vi "数据写入database.vi"(9 "data":variant, 10 "columns":string[](array[string]), 11 "table":string) -> (1 "error out":errorcluster)   [LabVIEW 2016, in "斯坦道CODMn.lvlib"]
uses:
  <vilib>/Utility/sysdir.llb/System Directory Type.ctl
  <vilib>/Utility/error.llb/DialogType.ctl
  <vilib>/addons/database/Auxilliary.llb/DB Tools Transaction.ctl
  <vilib>/addons/database/Auxilliary.llb/DB Tools Isolation Level.ctl
  <vilib>/addons/database/Connection.llb/DB Tools Open Connec (String).vi
  <vilib>/addons/database/Connection.llb/Conn Execute.vi
  <vilib>/addons/database/Recordset.llb/Rec Destroy - Connection.vi
  <vilib>/addons/database/Recordset.llb/Rec Fetch Recordset Data (R).vi
  <vilib>/addons/database/Connection.llb/Conn Transaction.vi
  <vilib>/addons/database/NI_Database_API.lvlib
panel:
  out "为空？":bool
  in  "error in (no error)":errorcluster
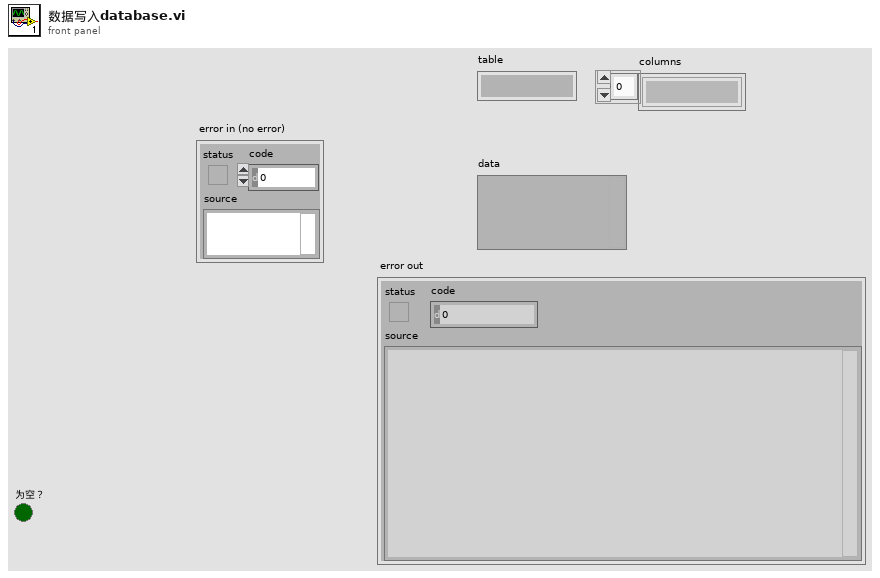
[diagram p1: front panel]
types:
  T1 = cluster{"时间":timestamp, "测量模式":string, "数据类型":string, "检测值":sgl, "单位":string, "数据标识":string, "因子编码":string, "标样参考值":sgl, "ORP-A":sgl, "ORP-B":sgl, "ORP-K":sgl, "COD滴定值":sgl, "高锰酸钾滴定数":sgl, "温度":sgl, "量程":sgl, "LastTime":timestamp, "序列号:":string}
  T2 = typedef "DialogType.ctl" = u16
  T3 = typedef "System Directory Type.ctl" = i32
  T4 = typedef "NI_Database_API.lvlib/Conn ObjectReference.ctl" = refnum<k1>
  T5 = typedef "NI_Database_API.lvlib/Rec ObjectReference.ctl" = refnum<k1>
  T6 = typedef "NI_Database_API.lvlib/DB Tools Transaction.ctl" = enum16{"begin", "commit", "rollback"}
  T7 = typedef "NI_Database_API.lvlib/DB Tools Isolation Level.ctl" = enum16{"chaos", "read uncommitted", "read committed", "repeatable read", "serializable"}
  T8 = cluster{"测量量程":dbl, "测量精度":dbl, "测量间隔":dbl, "消解温度":dbl, "消解时长":dbl, "空白校准时间":timestamp, "曲线截距":dbl, "曲线斜率":dbl, "测量检出限":dbl, "测量信号值":dbl, "线性相关系数":dbl, "二次多项式系数":dbl, "标样校准时间":timestamp, "稀释倍数":dbl, "三项式系数":dbl, "空白标定系数":dbl, "量程系数":dbl, "F0/ORPA":dbl, "F1/ORPB":dbl, "F2/ORPK":dbl, "F3":dbl, "F4":dbl, "F5":dbl, "F6":dbl, "F7":dbl, "X0/滴定数":dbl, "量程":dbl}
  T9 = cluster{"时间标识":timestamp, "设备":string, "日志信息":string}
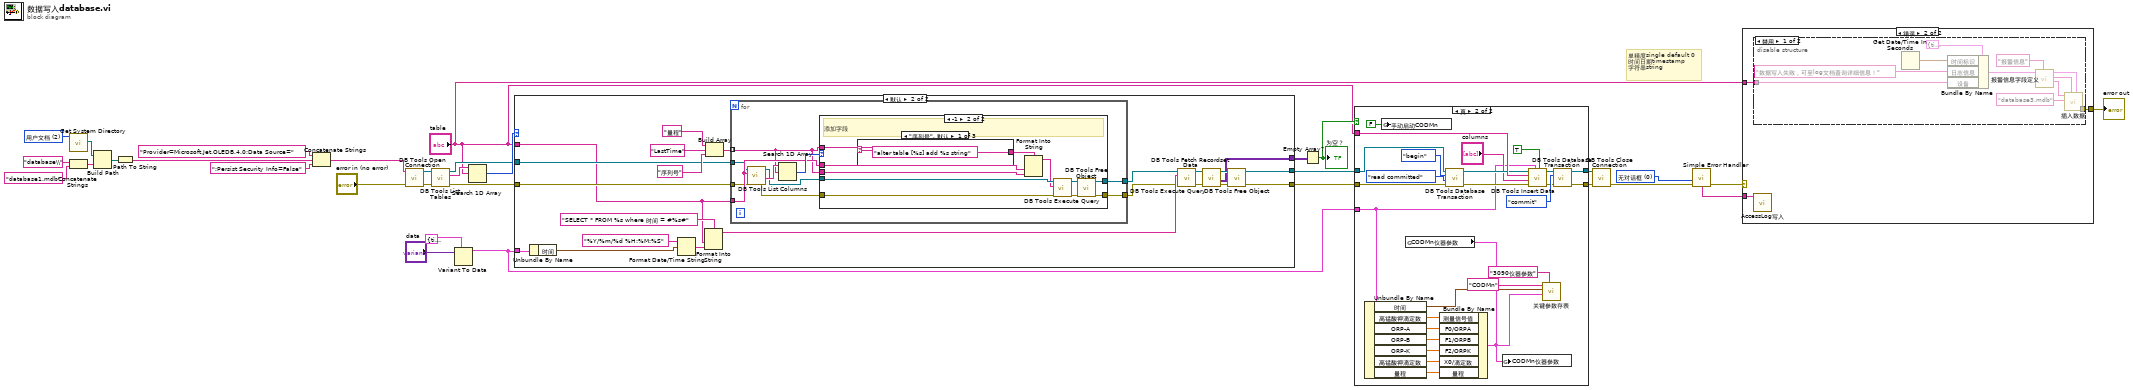
[diagram p0: block diagram]
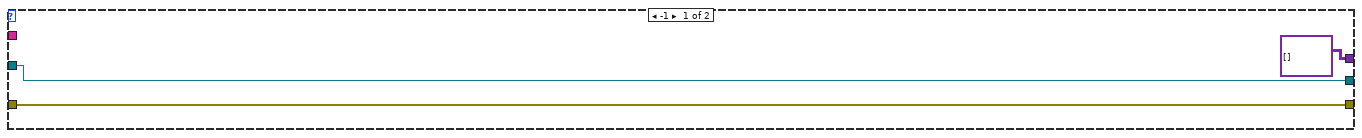
[diagram p4: hidden frame]
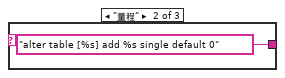
[diagram p6: hidden frame]
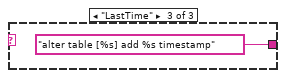
[diagram p7: hidden frame]
diagram:
  w8 = T2 0 items=["无对话框", "确定信息", "继续或停止信息", "确定信息＋警告", "继续/停止+警告"] ("type of dialog (OK msg:1)")
  w32 = T3 2 items=["用户目录"=0, "用户桌面"=1, "用户文档"=2, "用户应用程序数据"=3, "用户设置"=4, "用户临时目录"=5, "公共文档"=6, "公共应用程序数据"=7, "公共设置"=8, "公共缓存"=13, "系统核心库"=9, "系统安装库"=10, "应用程序文件"=11, "启动盘根目录"=12] ("system directory type")
  # "单精度single default 0\n时间日期timestamp\n字符串string"
  n1 = call <vilib>:"Get System Directory.vi"("system directory type"=w32) -> ("system directory"=w30:path)  [unwired: 10 in]
  n2 = Concatenate Strings("database\\" ("condition"), "database1.mdb" ("字符串")) -> (w24:string)
  n3 = Build Path(base path=w30, name or relative path=w24) -> (appended path=w29:path)
  n4 = Path To String(path=w29) -> (string=w28:string)
  n5 = Concatenate Strings("Provider=Microsoft.Jet.OLEDB.4.0;Data Source=" ("condition"), w28, ";Persist Security Info=False" ("condition")) -> (w26:string)
  n6 = call-poly <vilib>:"DB Tools Open Connection.vi"("error in (no error)"="error in (no error)", "connection information"=w26) -> ("error out"=w22:errorcluster, "connection reference"=w23:T4)  [unwired: 6 in]
  n7 = call <vilib>:"DB Tools List Tables.vi"("error in (no error)"=w22, "connection reference"=w23) -> ("error out"=w16:errorcluster, "tables"=w21:string[], "connection reference out"=w17:T4)  [unwired: 3 in]
  n8 = Variant To Data(type=T1 {"时间"=timestamp(0 s since 1904-01-01), "测量模式"="", "数据类型"="", "检测值"=0.0, "单位"="", "数据标识"="", "因子编码"="", "标样参考值"=0.0, "ORP-A"=0.0, "ORP-B"=0.0, "ORP-K"=0.0, "COD滴定值"=0.0, "高锰酸钾滴定数"=0.0, "温度"=0.0, "量程"=0.0, "LastTime"=timestamp(0 s since 1904-01-01), "序列号:"=""} ("data"), Variant="data") -> (data=w9:T1)  [unwired: 1 in, 1 out]
  n9 = Search 1D Array(1D array=w21, element="table") -> (index of element=w18:i32)  [unwired: 1 in]
  n10 = case shown="默认" w18 {
    tunnel: [variant[][] [] ("recordset data") w46] -> w15
    tunnel: [w35 w53] -> w14
    tunnel: [w34 w52] -> w13
    tunnel: w17 -> [w35 w40]
    tunnel: w16 -> [w34 w39]
    tunnel: "table" -> [_ w38]
    tunnel: w9 -> [_ w47]
    frame -1 {
    }
    frame Default {
      n11 = Unbundle By Name(w47) -> ("时间"=w50:timestamp)
      n12 = Format Date/Time String(time format string (%c)="%Y/%m/%d %H:%M:%S" ("时间格式字符串(%c)"), seconds (now)=w50) -> (date/time string=w48:string)  [unwired: 1 in]
      n13 = Format Into String(format string="SELECT * FROM %s where 时间 = #%s#" ("格式字符串"), w38, w48) -> (resulting string=w51:string)  [unwired: 2 in, 1 out]
      n14 = Build Array("量程" ("元素"), "LastTime" ("元素"), "序列号" ("元素")) -> (w44:string[])
      n15 = for {
        tunnel: w38 -> [w65]
        tunnel: w44 -> [w62] mode=indexing
        tunnel: [w61] -> w37
        tunnel: [w60] -> w36
        tunnel: w40 -> [w59]
        tunnel: w39 -> [w58]
        n16 = call <vilib>:"DB Tools List Columns.vi"("error in (no error)"=w58, "table"=w65, "connection reference"=w59) -> ("error out"=w63:errorcluster, "columns"=w67:string[], "connection reference out"=w64:T4)  [unwired: 1 in, 1 out]
        n17 = Search 1D Array(1D array=w67, element=w62) -> (index of element=w66:i32)  [unwired: 1 in]
        n18 = case shown="-1" w66 {
          tunnel: w64 -> [w69 w78]
          tunnel: w63 -> [w68 w77]
          tunnel: w62 -> [_ w76]
          tunnel: [w69 w74] -> w61
          tunnel: [w68 w73] -> w60
          tunnel: w65 -> [_ w72]
          tunnel: w62 -> [_ w71]
          frame 0, Default {
          }
          frame -1 {
            # "添加字段"
            n19 = case shown="\"序列号\", 默认" w71 {
              tunnel: ["alter table [%s] add %s string" "alter table [%s] add %s single default 0" "alter table [%s] add %s timestamp"] -> w70
              frame "序列号", Default {
              }
              frame "量程" {
              }
              frame "LastTime" {
              }
            }
            n20 = Format Into String(format string=w70, w72, w76) -> (resulting string=w75:string)  [unwired: 2 in, 1 out]
            n21 = call-poly <vilib>:"DB Tools Execute Query.vi"("error in (no error)"=w77, "SQL query"=w75, "connection reference"=w78) -> ("error out"=w79:errorcluster, "recordset reference"=w80:T5)  [unwired: 5 in]
            n22 = call-poly <vilib>:"DB Tools Free Object.vi"("error in (no error)"=w79, "recordset reference"=w80) -> ("error out"=w73:errorcluster, "connection reference"=w74:T4)  [unwired: 8 in]
          }
        }
      }
      n23 = call-poly <vilib>:"DB Tools Execute Query.vi"("error in (no error)"=w36, "SQL query"=w51, "connection reference"=w37) -> ("error out"=w54:errorcluster, "recordset reference"=w57:T5)  [unwired: 5 in]
      n24 = call-poly <vilib>:"DB Tools Fetch Recordset Data.vi"("error in (no error)"=w54, "recordset reference"=w57) -> ("error out"=w55:errorcluster, "recordset data"=w46:variant[][], "recordset reference out"=w56:T5)  [unwired: 3 in]
      n25 = call-poly <vilib>:"DB Tools Free Object.vi"("error in (no error)"=w55, "recordset reference"=w56) -> ("error out"=w52:errorcluster, "connection reference"=w53:T4)  [unwired: 8 in]
    }
  }
  n26 = Empty Array?(array=w15) -> (empty?=w10:bool)
  "为空？" <- w10
  n27 = case shown="真" w10 {
    tunnel: "table" -> [_ w111]
    tunnel: w9 -> [_ w96]
    tunnel: w13 -> [w84 w105]
    tunnel: w14 -> [w85 w106]
    tunnel: [w85 w100] -> w20
    tunnel: [w84 w99] -> w19
    frame False {
    }
    frame True {
      n28 = Unbundle By Name(w96) -> ("时间"=w94:timestamp, "高锰酸钾滴定数"=w95:sgl, "ORP-A"=w91:sgl, "ORP-B"=w90:sgl, "ORP-K"=w89:sgl, "高锰酸钾滴定数"=w87:sgl, "量程"=w86:sgl)
      n29 = global write "CODMN外部API.vi" "手动启动CODMn"(FALSE ("手动启动CODMn")) -> ()
      n30 = global read "CODMn断电保存全局变量.vi" "CODMn仪器参数"() -> (w97:T8)
      n31 = Bundle By Name(cluster=w97, "测量信号值"=w95, "F0/ORPA"=w91, "F1/ORPB"=w90, "F2/ORPK"=w89, "X0/滴定数"=w87, "量程"=w86) -> (w92:T8)
      n32 = call-poly <vilib>:"DB Tools Database Transaction.vi"("error in (no error)"=w105, "isolation level (chaos)"=DB_Tools_Isolation_Level."read committed", "operation (begin)"=DB_Tools_Transaction."begin", "connection reference"=w106) -> ("error out"=w103:errorcluster, "connection reference out"=w104:T4)  [unwired: 2 in]
      n33 = global write "CODMn断电保存全局变量.vi" "CODMn仪器参数"(w92) -> ()
      n34 = call <vilib>:"DB Tools Insert Data.vi"("create table? (F)"=TRUE, "data"=w96, "error in (no error)"=w103, "columns"="columns", "table"=w111, "connection reference"=w104) -> ("error out"=w101:errorcluster, "connection reference out"=w102:T4)  [unwired: 4 in]
      n35 = call "关键参数存表.vi"("table"="3090仪器参数", "仪器参数"=w92, "datatime"=w94, "仪器名称"="CODMn") -> ()  [unwired: 7 in, 1 out]
      n36 = call-poly <vilib>:"DB Tools Database Transaction.vi"("error in (no error)"=w101, "operation (begin)"=DB_Tools_Transaction."commit", "connection reference"=w102) -> ("error out"=w99:errorcluster, "connection reference out"=w100:T4)  [unwired: 3 in]
    }
  }
  n37 = call <vilib>:"DB Tools Close Connection.vi"("error in (no error)"=w19, "connection reference"=w20) -> ("error out"=w6:errorcluster)  [unwired: 5 in]
  n38 = call <vilib>:"Simple Error Handler.vi"("type of dialog (OK msg:1)"=w8, "error in (no error)"=w6) -> ("error out"=w7:errorcluster, "message"=w3:string)  [unwired: 3 in, 3 out]
  n39 = case shown="错误" w7 {
    tunnel: "table" -> [_ w115]
    tunnel: [_ w114] -> w4
    tunnel: w3 -> [_ w113]
    frame No Error {
    }
    frame Error {
      n40 = call "AccessLog写入.vi"("Log"=w113) -> ()  [unwired: 11 in]
      n41 = disable-structure shown="禁用" {
        disable-tunnel: w115 -> [w124 _]
        disable-tunnel: [w117 _] -> w114
        frame Disabled {
          n42 = Get Date/Time In Seconds() -> (seconds since 1Jan1904=w125:timestamp)
          n43 = Bundle By Name(cluster=T9 {"时间标识"=timestamp(0 s since 1904-01-01), "设备"="氨氮", "日志信息"=""} ("data in"), "时间标识"=w125, "日志信息"="数据写入失败，可至log文档查询详细信息！" ("table输入"), "设备"=w124) -> (w118:T9)
          n44 = call "报警信息字段定义.vi"("table输入"="报警信息", "data in"=w118) -> ("table输出"=w121:string, "columns"=w122:string[], "data out"=w123:T9)  [unwired: 7 in]
          n45 = call "插入数据.vi"("data"=w123, "columns"=w122, "database"="database3.mdb", "table"=w121) -> ("error out"=w117:errorcluster)  [unwired: 7 in]
        }
        frame Enabled {
        }
      }
    }
  }
  "error out" <- w4
